vi "Number of Pixels.vi"(11 "image data":T1) -> (3 "Number of Pixels":u64)   [LabVIEW 2014, in "Image Comparison.lvclass"]
uses:
  Image Comparison.lvclass
  <vilib>/picture/picture.llb/imagedata.ctl
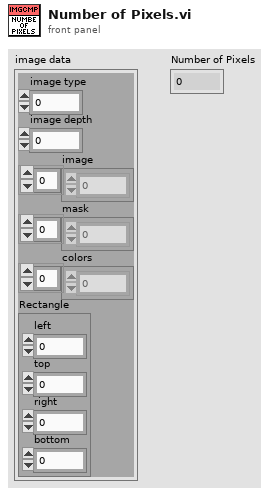
[diagram p1: front panel]
types:
  T1 = typedef "imagedata.ctl" = cluster{"image type":i32, "image depth":i32, "image":u8[], "mask":u8[], "colors":u32[], "Rectangle":cluster{"left":i16, "top":i16, "right":i16, "bottom":i16}}
  T2 = cluster{"left":i16, "top":i16, "right":i16, "bottom":i16}
  T3 = cluster{"left":u64, "top":u64, "right":u64, "bottom":u64}
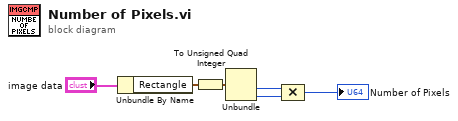
[diagram p0: block diagram]
diagram:
  n1 = Unbundle By Name("image data") -> ("Rectangle"=w5:T2)
  n2 = To Unsigned Quad Integer(1:w5) -> (0:w1:T3)
  n3 = Unbundle(w1) -> ("right"=w4:u64, "bottom"=w3:u64)  [unwired: 2 out]
  n4 = Compound Arithmetic op=MULTIPLY(w4, w3) -> (→"Number of Pixels":u64)
